vi "Write Manager UI References.vi"(8 "error in (no error)":errorcluster, 10 "Manager UI References":T1, 11 "CIF_UI in":refnum<class "CIF_Manager_UI.lvclass">) -> (0 "error out":errorcluster, 3 "CIF_UI out":refnum<class "CIF_Manager_UI.lvclass">)   [LabVIEW 2021, in "CIF_Manager_UI.lvclass"]
uses:
  CIF_Manager_UI.lvclass
  Typedef/Core Manager UI References.ctl
  Typedef/Channel Connection.ctl
  Typedef/New Plugin.ctl
  Typedef/CIF_Manager_UI_Tab.ctl
  CIF_Manager_UI.lvclass/CIF_Manager_UI.ctl
  <vilib>/CIF Foundation/CIF Core/CIFUI/Accessors/Read Instrument Studio.vi
  <vilib>/CIF Foundation/CIF Core/CIFUI/CIF_UI.lvclass
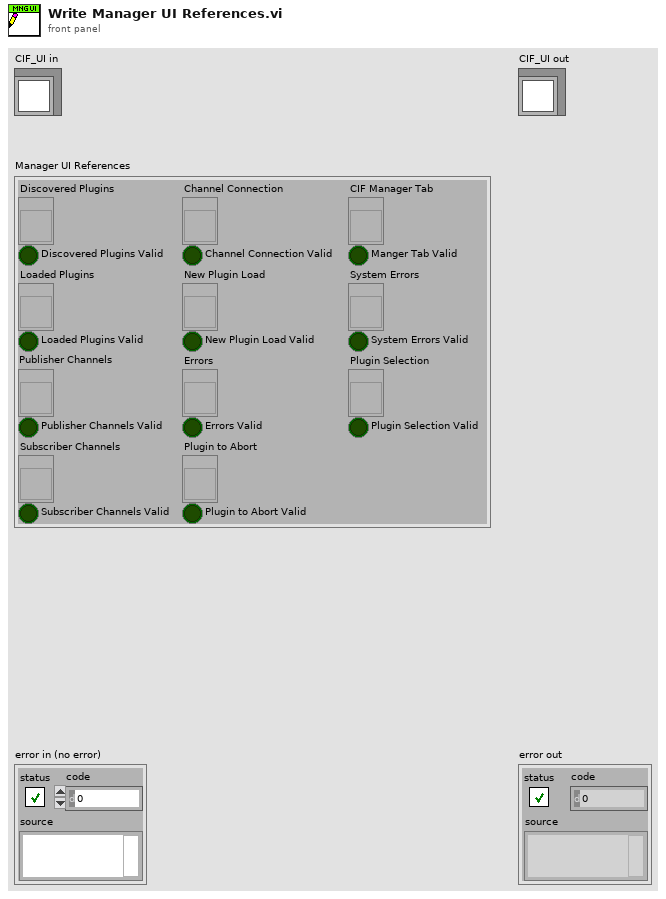
[diagram p1: front panel]
types:
  T1 = typedef "CIF_Manager_UI.lvclass/Core Manager UI References.ctl" = cluster{"Discovered Plugins":refnum<vi>, "Discovered Plugins Valid":bool, "Loaded Plugins":refnum<vi>, "Loaded Plugins Valid":bool, "Publisher Channels":refnum<vi>, "Publisher Channels Valid":bool, "Subscriber Channels":refnum<vi>, "Subscriber Channels Valid":bool, "Channel Connection":refnum<vi>, "Channel Connection Valid":bool, "New Plugin Load":refnum<vi>, "New Plugin Load Valid":bool, "Errors":refnum<vi>, "Errors Valid":bool, "Plugin to Abort":refnum<vi>, "Plugin to Abort Valid":bool, "CIF Manager Tab":refnum<vi>, "Manger Tab Valid":bool, "System Errors":refnum<vi>, "System Errors Valid":bool, "Plugin Selection":refnum<vi>, "Plugin Selection Valid":bool}
  T2 = typedef "CIF_Manager_UI.lvclass/Channel Connection.ctl" = cluster{"Publisher Name":string, "Subscriber Name":string, "Custom Data":string, "FIFO Overrides":cluster{"Backpressure":bool, "Bytes/Message":u32, "Messages/FIFO":u32}}
  T3 = typedef "CIF_Manager_UI.lvclass/New Plugin.ctl" = cluster{"Unique Name":string, "Type":string, "Version (Optional)":string, "Loader (Optional)":string}
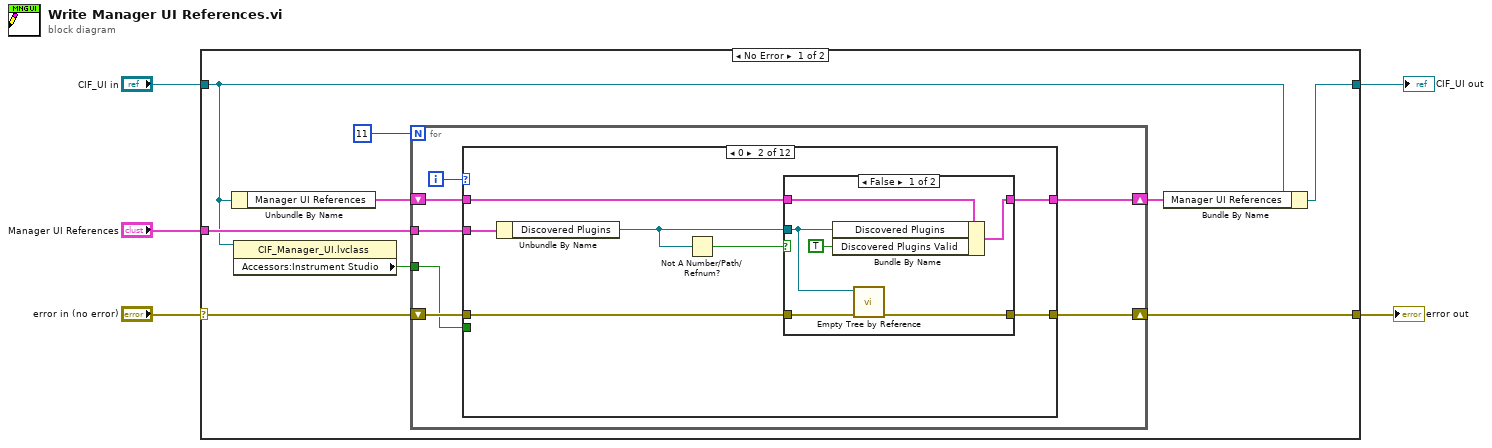
[diagram p0: block diagram]
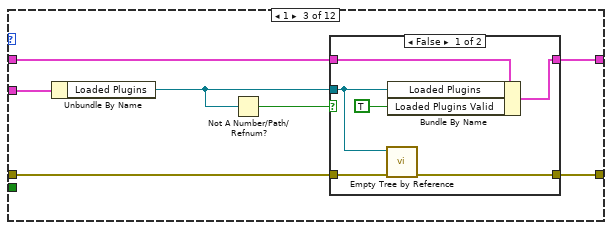
[diagram p4: hidden frame]
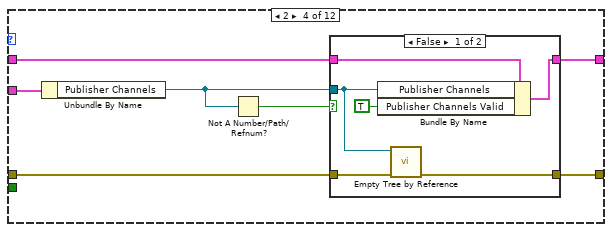
[diagram p6: hidden frame]
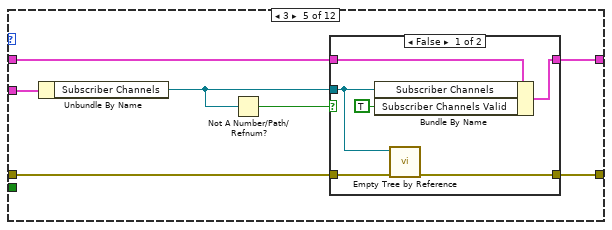
[diagram p8: hidden frame]
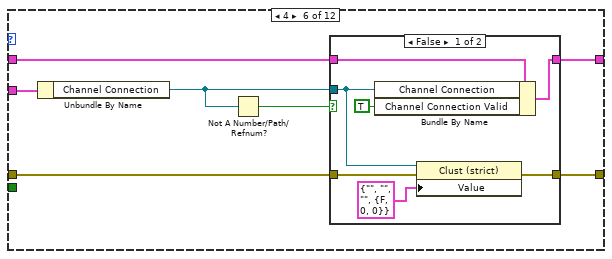
[diagram p10: hidden frame]
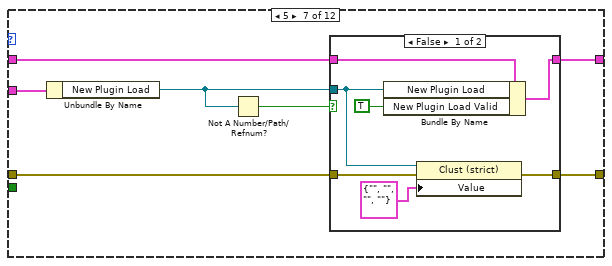
[diagram p12: hidden frame]
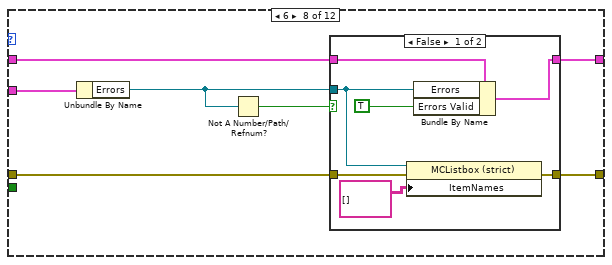
[diagram p14: hidden frame]
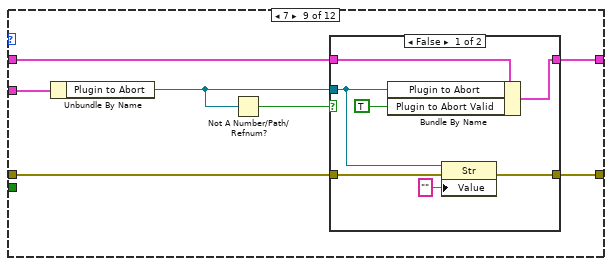
[diagram p16: hidden frame]
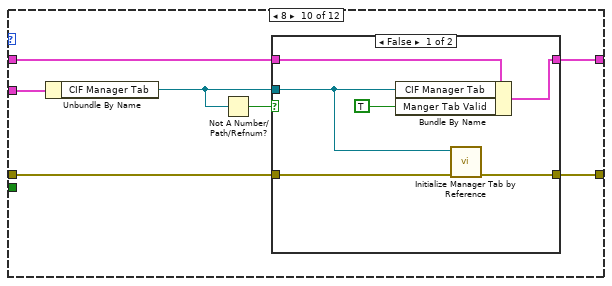
[diagram p18: hidden frame]
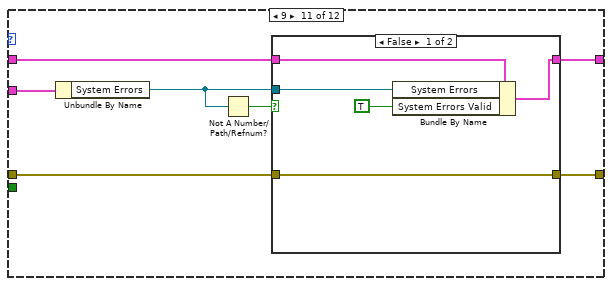
[diagram p20: hidden frame]
diagram:
  n1 = case shown="No Error" "error in (no error)" {
    selector: "error in (no error)" -> [w9 w191]
    tunnel: [w8 w191] -> w4
    tunnel: [w14 w192] -> w2
    tunnel: "CIF_UI in" -> [w7 w192]
    tunnel: "Manager UI References" -> [w13 _]
    frame No Error {
      n2 = Unbundle By Name(w7) -> ("Manager UI References"=w12:T1)
      n3 = property class="CIF_Manager_UI.lvclass"(reference=w7) -> ("Accessors:Instrument Studio"=w6:bool)  [unwired: 1 in, 2 out]
      n4 = for {
        N: 11 -> [_]
        shift-right: [w18] -> w11
        shift-left: w12 -> [w19]
        tunnel: w13 -> [w20]
        shift-right: [w16] -> w8
        shift-left: w9 -> [w17]
        tunnel: w6 -> [w15]
        i -> [w21]
        n5 = case shown="0" w21 {
          tunnel: w20 -> [_ w30 w45 w60 w75 w90 w106 w122 w138 w154 w169 w183]
          tunnel: w19 -> [w23 w29 w44 w59 w74 w89 w105 w121 w137 w153 w168 w182]
          tunnel: [w23 w28 w43 w58 w73 w88 w104 w120 w136 w152 w167 w181] -> w18
          tunnel: w17 -> [w22 w25 w40 w55 w70 w84 w100 w116 w132 w148 w163 w177]
          tunnel: [w22 w24 w39 w54 w69 w85 w101 w117 w133 w149 w164 w178] -> w16
          tunnel: w15 -> [_ _ _ _ _ _ _ _ _ _ _ _]
          frame -1, Default {
          }
          frame 0 {
            n6 = Unbundle By Name(w30) -> ("Discovered Plugins"=w27:refnum<vi>)
            n7 = Not A Number/Path/Refnum?(number/path/refnum=w27) -> (NaN/Path/Refnum?=w26:bool)
            n8 = case shown="False" w26 {
              tunnel: w27 -> [w33 _]
              tunnel: w29 -> [w36 w38]
              tunnel: [w35 w38] -> w28
              tunnel: w25 -> [w32 w37]
              tunnel: [w31 w37] -> w24
              frame False {
                n9 = Bundle By Name(cluster=w36, "Discovered Plugins"=w33, "Discovered Plugins Valid"=TRUE) -> (w35:T1)
                n10 = call <vilib>:"Empty Tree by Reference.vi"("error in (no error)"=w32, "Tree ref in"=w33) -> ("error out"=w31:errorcluster)  [unwired: 9 in]
              }
              frame True {
              }
            }
          }
          frame 1 {
            n11 = Unbundle By Name(w45) -> ("Loaded Plugins"=w42:refnum<vi>)
            n12 = Not A Number/Path/Refnum?(number/path/refnum=w42) -> (NaN/Path/Refnum?=w41:bool)
            n13 = case shown="False" w41 {
              tunnel: w42 -> [w48 _]
              tunnel: w44 -> [w51 w53]
              tunnel: [w50 w53] -> w43
              tunnel: w40 -> [w47 w52]
              tunnel: [w46 w52] -> w39
              frame False {
                n14 = call <vilib>:"Empty Tree by Reference.vi"("error in (no error)"=w47, "Tree ref in"=w48) -> ("error out"=w46:errorcluster)  [unwired: 9 in]
                n15 = Bundle By Name(cluster=w51, "Loaded Plugins"=w48, "Loaded Plugins Valid"=TRUE ("Discovered Plugins Valid")) -> (w50:T1)
              }
              frame True {
              }
            }
          }
          frame 2 {
            n16 = Unbundle By Name(w60) -> ("Publisher Channels"=w57:refnum<vi>)
            n17 = Not A Number/Path/Refnum?(number/path/refnum=w57) -> (NaN/Path/Refnum?=w56:bool)
            n18 = case shown="False" w56 {
              tunnel: w57 -> [w62 _]
              tunnel: w59 -> [w66 w68]
              tunnel: [w65 w68] -> w58
              tunnel: w55 -> [w63 w67]
              tunnel: [w61 w67] -> w54
              frame False {
                n19 = Bundle By Name(cluster=w66, "Publisher Channels"=w62, "Publisher Channels Valid"=TRUE ("Discovered Plugins Valid")) -> (w65:T1)
                n20 = call <vilib>:"Empty Tree by Reference.vi"("error in (no error)"=w63, "Tree ref in"=w62) -> ("error out"=w61:errorcluster)  [unwired: 9 in]
              }
              frame True {
              }
            }
          }
          frame 3 {
            n21 = Unbundle By Name(w75) -> ("Subscriber Channels"=w72:refnum<vi>)
            n22 = Not A Number/Path/Refnum?(number/path/refnum=w72) -> (NaN/Path/Refnum?=w71:bool)
            n23 = case shown="False" w71 {
              tunnel: w72 -> [w78 _]
              tunnel: w74 -> [w81 w83]
              tunnel: [w80 w83] -> w73
              tunnel: w70 -> [w77 w82]
              tunnel: [w76 w82] -> w69
              frame False {
                n24 = Bundle By Name(cluster=w81, "Subscriber Channels"=w78, "Subscriber Channels Valid"=TRUE ("Discovered Plugins Valid")) -> (w80:T1)
                n25 = call <vilib>:"Empty Tree by Reference.vi"("error in (no error)"=w77, "Tree ref in"=w78) -> ("error out"=w76:errorcluster)  [unwired: 9 in]
              }
              frame True {
              }
            }
          }
          frame 4 {
            n26 = Unbundle By Name(w90) -> ("Channel Connection"=w87:refnum<vi>)
            n27 = Not A Number/Path/Refnum?(number/path/refnum=w87) -> (NaN/Path/Refnum?=w86:bool)
            n28 = case shown="False" w86 {
              tunnel: w87 -> [w94 _]
              tunnel: w89 -> [w97 w99]
              tunnel: [w96 w99] -> w88
              tunnel: [w93 w98] -> w85
              tunnel: w84 -> [w92 w98]
              frame False {
                n29 = Bundle By Name(cluster=w97, "Channel Connection"=w94, "Channel Connection Valid"=TRUE ("Discovered Plugins Valid")) -> (w96:T1)
                n30 = property on="Property Node" class="Clust (strict)"(reference=w94, error in=w92, "Value"=T2 {"Publisher Name"="", "Subscriber Name"="", "Custom Data"="", "FIFO Overrides"={"Backpressure"=FALSE, "Bytes/Message"=0, "Messages/FIFO"=0}}) -> (error out=w93:errorcluster)  [unwired: 1 out]
              }
              frame True {
              }
            }
          }
          frame 5 {
            n31 = Unbundle By Name(w106) -> ("New Plugin Load"=w103:refnum<vi>)
            n32 = Not A Number/Path/Refnum?(number/path/refnum=w103) -> (NaN/Path/Refnum?=w102:bool)
            n33 = case shown="False" w102 {
              tunnel: w103 -> [w110 _]
              tunnel: w105 -> [w113 w115]
              tunnel: [w112 w115] -> w104
              tunnel: [w109 w114] -> w101
              tunnel: w100 -> [w108 w114]
              frame False {
                n34 = Bundle By Name(cluster=w113, "New Plugin Load"=w110, "New Plugin Load Valid"=TRUE ("Discovered Plugins Valid")) -> (w112:T1)
                n35 = property on="Property Node" class="Clust (strict)"(reference=w110, error in=w108, "Value"=T3 {"Unique Name"="", "Type"="", "Version (Optional)"="", "Loader (Optional)"=""}) -> (error out=w109:errorcluster)  [unwired: 1 out]
              }
              frame True {
              }
            }
          }
          frame 6 {
            n36 = Unbundle By Name(w122) -> ("Errors"=w119:refnum<vi>)
            n37 = Not A Number/Path/Refnum?(number/path/refnum=w119) -> (NaN/Path/Refnum?=w118:bool)
            n38 = case shown="False" w118 {
              tunnel: w119 -> [w126 _]
              tunnel: w121 -> [w129 w131]
              tunnel: [w128 w131] -> w120
              tunnel: [w125 w130] -> w117
              tunnel: w116 -> [w124 w130]
              frame False {
                n39 = property on="Property Node" class="MCListbox (strict)"(reference=w126, error in=w124, "ItemNames"=string[][] [] ("Item Names")) -> (error out=w125:errorcluster)  [unwired: 1 out]
                n40 = Bundle By Name(cluster=w129, "Errors"=w126, "Errors Valid"=TRUE ("Discovered Plugins Valid")) -> (w128:T1)
              }
              frame True {
              }
            }
          }
          frame 7 {
            n41 = Unbundle By Name(w138) -> ("Plugin to Abort"=w135:refnum<vi>)
            n42 = Not A Number/Path/Refnum?(number/path/refnum=w135) -> (NaN/Path/Refnum?=w134:bool)
            n43 = case shown="False" w134 {
              tunnel: w135 -> [w142 _]
              tunnel: w137 -> [w145 w147]
              tunnel: [w144 w147] -> w136
              tunnel: [w141 w146] -> w133
              tunnel: w132 -> [w140 w146]
              frame False {
                n44 = Bundle By Name(cluster=w145, "Plugin to Abort"=w142, "Plugin to Abort Valid"=TRUE ("Discovered Plugins Valid")) -> (w144:T1)
                n45 = property on="Property Node" class="Str"(reference=w142, error in=w140, "Value"="") -> (error out=w141:errorcluster)  [unwired: 1 out]
              }
              frame True {
              }
            }
          }
          frame 8 {
            n46 = Unbundle By Name(w154) -> ("CIF Manager Tab"=w151:refnum<vi>)
            n47 = Not A Number/Path/Refnum?(number/path/refnum=w151) -> (NaN/Path/Refnum?=w150:bool)
            n48 = case shown="False" w150 {
              tunnel: w151 -> [w155 _]
              tunnel: w153 -> [w160 w162]
              tunnel: [w159 w162] -> w152
              tunnel: [w156 w161] -> w149
              tunnel: w148 -> [w157 w161]
              frame False {
                n49 = Bundle By Name(cluster=w160, "CIF Manager Tab"=w155, "Manger Tab Valid"=TRUE ("Discovered Plugins Valid")) -> (w159:T1)
                n50 = call "Initialize Manager Tab by Reference.vi"("error in (no error)"=w157, "CIF Manager UI Tab"=w155) -> ("error out"=w156:errorcluster)  [unwired: 9 in]
              }
              frame True {
              }
            }
          }
          frame 9 {
            n51 = Unbundle By Name(w169) -> ("System Errors"=w166:refnum<vi>)
            n52 = Not A Number/Path/Refnum?(number/path/refnum=w166) -> (NaN/Path/Refnum?=w165:bool)
            n53 = case shown="False" w165 {
              tunnel: w166 -> [w171 _]
              tunnel: w168 -> [w174 w176]
              tunnel: [w173 w176] -> w167
              tunnel: [w170 w175] -> w164
              tunnel: w163 -> [w170 w175]
              frame False {
                n54 = Bundle By Name(cluster=w174, "System Errors"=w171, "System Errors Valid"=TRUE ("Discovered Plugins Valid")) -> (w173:T1)
              }
              frame True {
              }
            }
          }
          frame 10 {
            n55 = Unbundle By Name(w183) -> ("Plugin Selection"=w180:refnum<vi>)
            n56 = Not A Number/Path/Refnum?(number/path/refnum=w180) -> (NaN/Path/Refnum?=w179:bool)
            n57 = case shown="False" w179 {
              tunnel: w180 -> [w185 _]
              tunnel: w182 -> [w188 w190]
              tunnel: [w187 w190] -> w181
              tunnel: [w184 w189] -> w178
              tunnel: w177 -> [w184 w189]
              frame False {
                n58 = Bundle By Name(cluster=w188, "Plugin Selection"=w185, "Plugin Selection Valid"=TRUE ("Discovered Plugins Valid")) -> (w187:T1)
              }
              frame True {
              }
            }
          }
        }
      }
      n59 = Bundle By Name(cluster=w7, "Manager UI References"=w11) -> (w14:refnum<class "CIF_Manager_UI.lvclass">)
    }
    frame Error {
    }
  }
  "error out" <- w4
  "CIF_UI out" <- w2
